vi "_wmg_readFile.vi"(1 "路径":path) -> (0 "字符串":string)   [LabVIEW 2011]
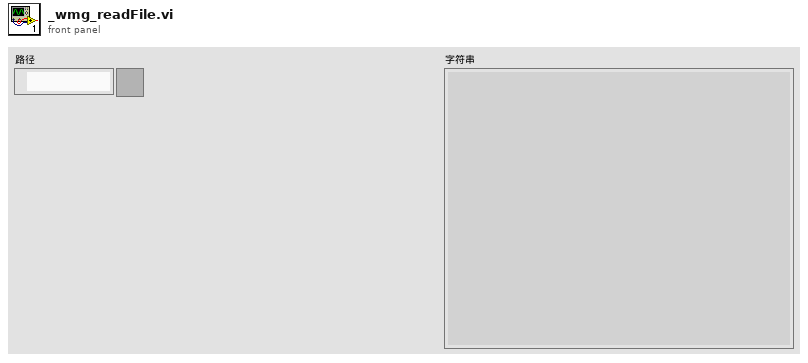
[diagram p1: front panel]
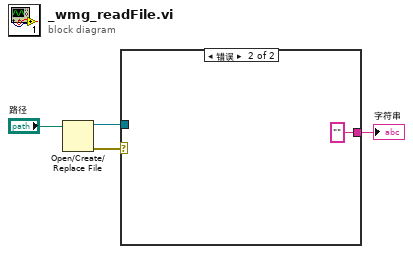
[diagram p0: block diagram]
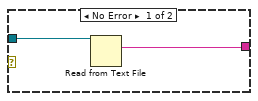
[diagram p2: hidden frame]
diagram:
  n1 = Open/Create/Replace File(file path (use dialog)="路径") -> (refnum out=w1:refnum<file>, error out=w3:errorcluster)  [unwired: 5 in, 1 out]
  n2 = case shown="错误" w3 {
    tunnel: [w5 ""] -> w2
    tunnel: w1 -> [w6 _]
    frame No Error {
      n3 = Read from Text File(file (use dialog)=w6) -> (text=w5:string)  [unwired: 3 in, 3 out]
    }
    frame Error {
    }
  }
  "字符串" <- w2
